vi "Read Tail.vi"(8 "error in (no error)":errorcluster, 11 "CIPC Reference":u64) -> (0 "error out":errorcluster, 3 "Tail":u32)   [LabVIEW 2021, in "CIF_NI_CIPC.lvlib"]
uses:
  CIF_NI_CIPC.lvlib
  <vilib>/Utility/error.llb/Trim Whitespace.vi
  <vilib>/Utility/error.llb/Error Cluster From Error Code.vi
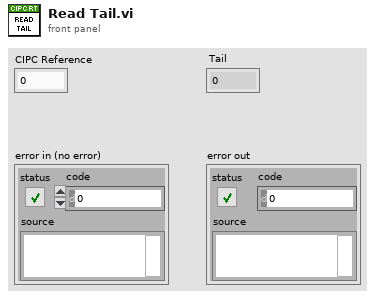
[diagram p1: front panel]
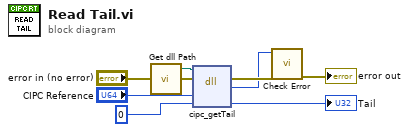
[diagram p0: block diagram]
diagram:
  n1 = call "Get dll Path.vi"() -> ("appended path"=w1:path)  [unwired: 5 in]
  n2 = dll-call lib="libnicipc.*" fn="cipc_getTail"(path in=w1, error in="error in (no error)", "cipc_buffer_ref"="CIPC Reference", "tail"=u32 0 ("head")) -> (error out=w7:errorcluster, "return type"=w6:i32, "tail"=→"Tail":u32)  [unwired: 2 in, 1 out]
  n3 = call "Check Error.vi"("error in (no error)"=w7, "Error Code"=w6) -> ("error out"=→"error out":errorcluster)  [unwired: 9 in]
